vi "USB - Send Initialization Command to DAQ.vi"(8 "error in":errorcluster, 11 "VISA resource name in":refnum<visa-resource-name>) -> (0 "error out":errorcluster, 3 "VISA resource name out":refnum<visa-resource-name>)   [LabVIEW 2021]
doc: "Send a series of commands to initialize the DAQ device.\nTurn echo on, stop any data streaming, set power state, set data format to JSON."
uses:
  <vilib>/Instr/_visa.llb/VISA Flush IO Buffer Mask.ctl
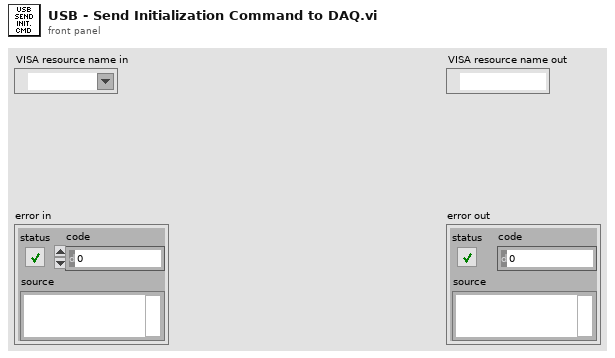
[diagram p1: front panel]
types:
  T1 = typedef "VISA Flush IO Buffer Mask.ctl" = u16
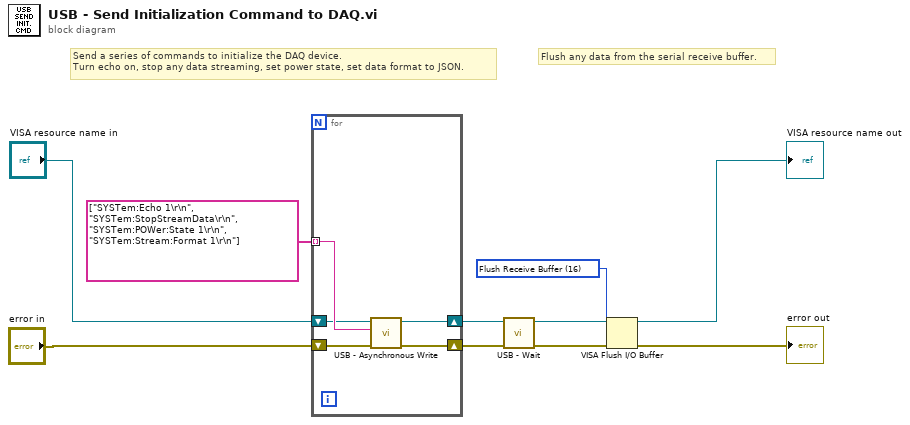
[diagram p0: block diagram]
diagram:
  w1 = T1 16 items=["Flush Receive Buffer"=16, "Write Transmit Buffer to Device"=32, "Flush Receive Buffer (No I/O)"=64, "Flush Transmit Buffer"=128] ("Mask")
  # "Flush any data from the serial receive buffer."
  # "Send a series of commands to initialize the DAQ device.\nTurn echo on, stop any data streaming, set power state, set data format to JSON."
  n1 = for {
    tunnel: string[] ["SYSTem:Echo 1\r\n", "SYSTem:StopStreamData\r\n", "SYSTem:POWer:State 1\r\n", "SYSTem:Stream:Format 1\r\n"] ("Array of Messages to Send") -> [w14] mode=indexing
    shift-right: [w12] -> w6
    shift-left: "VISA resource name in" -> [w13]
    shift-right: [w11] -> w5
    shift-left: "error in" -> [w15]
    n2 = call "USB - Asynchronous Write.vi"("error in"=w15, "Message to Send"=w14, "VISA resource name in"=w13) -> ("error out"=w11:errorcluster, "VISA resource name out"=w12:refnum<visa-resource-name>)  [unwired: 7 in]
  }
  n3 = call "USB - Wait.vi"("error in"=w5, "VISA Resource Name In"=w6) -> ("error out"=w4:errorcluster, "VISA Resource Name Out"=w7:refnum<visa-resource-name>)  [unwired: 8 in]
  n4 = VISA Flush I/O Buffer(VISA resource name=w7, mask (16)=w1, error in (no error)=w4) -> (VISA resource name out=→"VISA resource name out":refnum<visa-resource-name>, error out=→"error out":errorcluster)
